vi "SDG60LoadPolarity.vi"(0 "VISA resource name":refnum<visa-resource-name>="USB0::0xF4EC::0x1101::SDG6XEBC5R0119::INSTR", 1 "Channel (1: Channel1)":u16(ring)=1 items=["Channel1"=1, "Channel2"=2], 2 "Impedance (50.0 Ohms)":dbl=50.0 format="%#_15g", 3 "error in (no error)":errorcluster, 4 "Polarity (0: Normal)":u16(ring) items=["Normal", "Inverted"]) -> (5 "VISA resource name out":refnum<visa-resource-name>, 6 "error out":errorcluster)   [LabVIEW 2018]
doc: "Configures the output impedance and source impedance for the channel you specify."
panel:
  # "50..100K, or HiZ if larger"
  # "Changing impedance changes the\nset amplitude to maintain the same output amplitued"
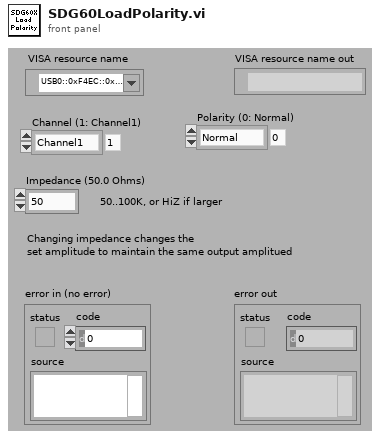
[diagram p1: front panel]
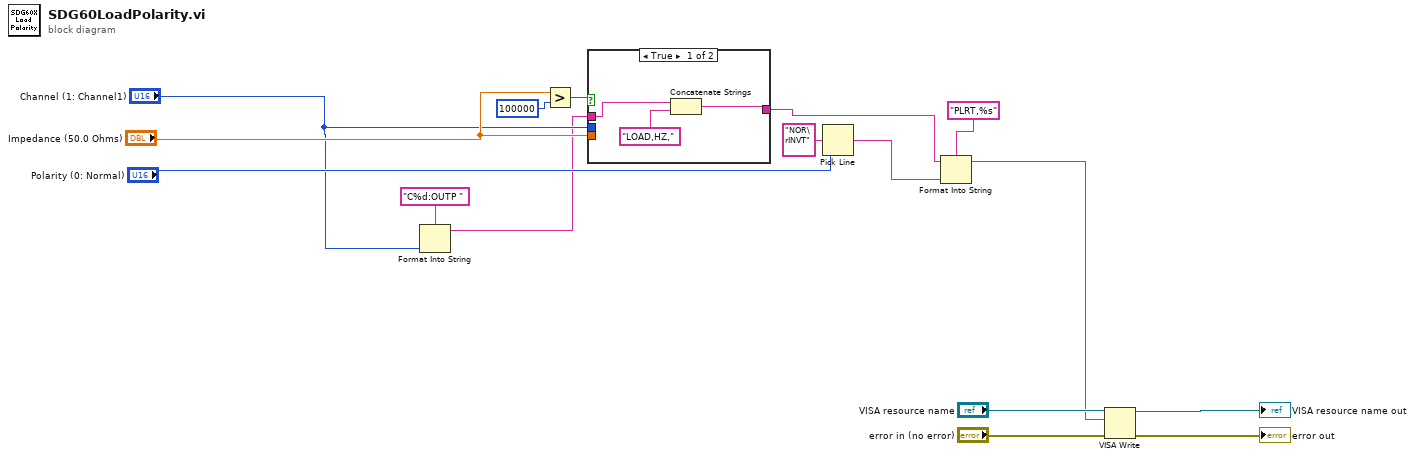
[diagram p0: block diagram]
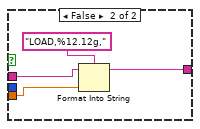
[diagram p2: hidden frame]
diagram:
  n1 = Format Into String(format string="C%d:OUTP ", "Channel (1: Channel1)") -> (resulting string=w1:string)  [unwired: 2 in, 1 out]
  n2 = Greater?(x="Impedance (50.0 Ohms)", y=100000) -> (0:w6:bool)
  n3 = case shown="True" w6 {
    tunnel: "Impedance (50.0 Ohms)" -> [_ w20]
    tunnel: [w17 w22] -> w9
    tunnel: "Channel (1: Channel1)" -> [_ _]
    tunnel: w1 -> [w18 w21]
    frame True {
      n4 = Concatenate Strings(w18, "LOAD,HZ,") -> (w17:string)
    }
    frame False {
      n5 = Format Into String(format string="LOAD,%12.12g,", initial string=w21, w20) -> (resulting string=w22:string)  [unwired: 1 in, 1 out]
    }
  }
  n6 = Pick Line(multi-line string="NOR\rINVT", line index="Polarity (0: Normal)") -> (output string=w5:string)  [unwired: 1 in]
  n7 = Format Into String(format string="PLRT,%s", initial string=w9, w5) -> (resulting string=w4:string)  [unwired: 1 in, 1 out]
  n8 = VISA Write(VISA resource name="VISA resource name", write buffer=w4, error in (no error)="error in (no error)") -> (VISA resource name out=→"VISA resource name out":refnum<visa-resource-name>, error out=→"error out":errorcluster)  [unwired: 1 out]
